vi "24vRelay_Powerstage_v1.vi"() -> (3 "Pass/Fail":bool)   [LabVIEW 2022 SP3]
uses:
  <vilib>/DAQmx/read.llb/DAQmx Read (Digital 1D Bool NChan 1Samp 1Line).vi
  <vilib>/DAQmx/miscellaneous.llb/DAQmx Fill In Error Info.vi
panel:
  out "error out":errorcluster
  out "data":bool[](array[boolean])
  in  "error in (no error)":errorcluster
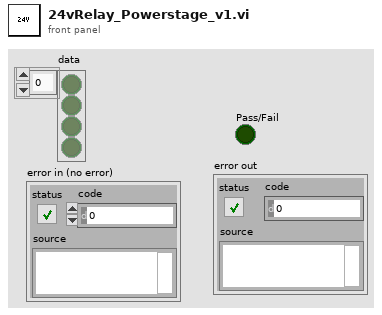
[diagram p1: front panel]
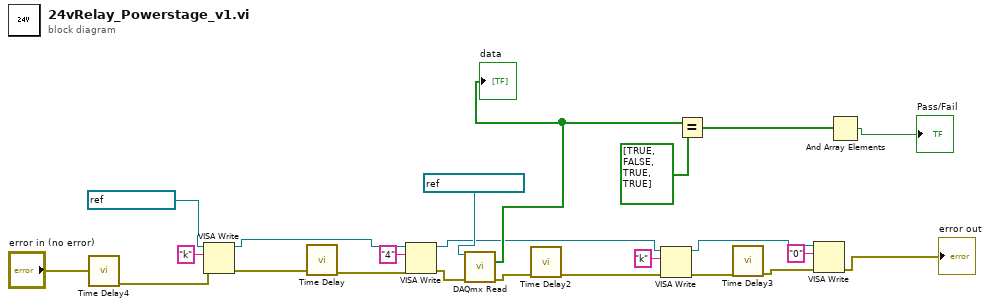
[diagram p0: block diagram]
diagram:
  n1 = call "Time Delay4"("error in (no error)"="error in (no error)") -> ("error out"=w1:errorcluster)  [unwired: 10 in]
  n2 = VISA Write(VISA resource name=refnum<visa-resource-name> "ControlBoard", write buffer="k", error in (no error)=w1) -> (VISA resource name out=w19:refnum<visa-resource-name>, error out=w21:errorcluster)  [unwired: 1 out]
  n3 = call "Time Delay"("error in (no error)"=w21) -> ("error out"=w20:errorcluster)  [unwired: 10 in]
  n4 = VISA Write(VISA resource name=w19, write buffer="4", error in (no error)=w20) -> (VISA resource name out=w3:refnum<visa-resource-name>, error out=w11:errorcluster)  [unwired: 1 out]
  n5 = call-poly <vilib>:"DAQmx Read.vi"("task/channels in"=refnum<k21> "FTS2_DigitalIn", "error in"=w11) -> ("data"=w8:bool[], "error out"=w10:errorcluster)  [unwired: 11 in, 1 out]
  "data" <- w8
  n6 = call "Time Delay2"("error in (no error)"=w10) -> ("error out"=w17:errorcluster)  [unwired: 10 in]
  n7 = VISA Write(VISA resource name=w3, write buffer="k", error in (no error)=w17) -> (VISA resource name out=w14:refnum<visa-resource-name>, error out=w16:errorcluster)  [unwired: 1 out]
  n8 = Equal?(x=w8, y=bool[] [TRUE, FALSE, TRUE, TRUE]) -> (x = y?=w6:bool[])
  n9 = call "Time Delay3"("error in (no error)"=w16) -> ("error out"=w15:errorcluster)  [unwired: 10 in]
  n10 = VISA Write(VISA resource name=w14, write buffer="0", error in (no error)=w15) -> (error out=→"error out":errorcluster)  [unwired: 2 out]
  n11 = And Array Elements(Boolean array=w6) -> (logical AND=→"Pass/Fail":bool)
